vi "initializer_set_time.vi"(6 "Parameters Tree":refnum<vi>, 9 "Endtime":refnum<vi>, 10 "Starttime":refnum<vi>, 11 "Spec File Loaded?":refnum<vi>) -> ()   [LabVIEW 2019]
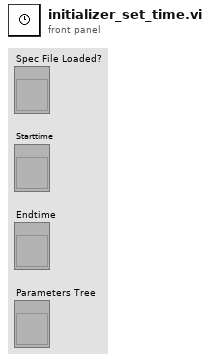
[diagram p1: front panel]
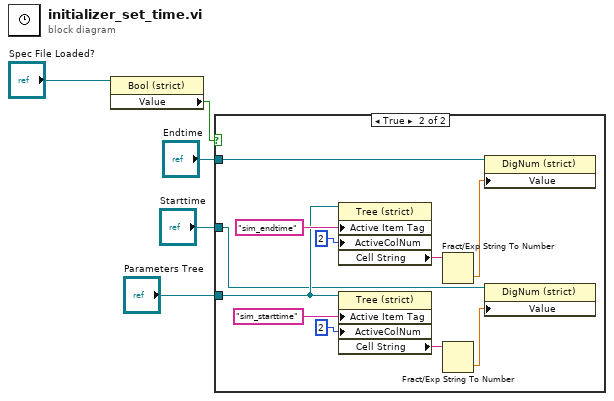
[diagram p0: block diagram]
diagram:
  n1 = property class="Bool (strict)"(reference="Spec File Loaded?") -> ("Value"=w5:bool)  [unwired: 1 in, 2 out]
  n2 = case shown="True" w5 {
    tunnel: "Parameters Tree" -> [_ w12]
    tunnel: "Starttime" -> [_ w7]
    tunnel: "Endtime" -> [_ w6]
    frame False {
    }
    frame True {
      n3 = property on="Property Node" class="Tree (strict)"(reference=w12, "Active Item Tag"="sim_endtime" ("Active Item:Tag"), "ActiveColNum"=2 ("Active Cell:Active Column Number")) -> ("Cell String"=w11:string)  [unwired: 1 in, 2 out]
      n4 = property on="Property Node" class="Tree (strict)"(reference=w12, "Active Item Tag"="sim_starttime" ("Active Item:Tag"), "ActiveColNum"=2 ("Active Cell:Active Column Number")) -> ("Cell String"=w10:string)  [unwired: 1 in, 2 out]
      n5 = Fract/Exp String To Number(string=w11) -> (number=w8:dbl)  [unwired: 3 in, 1 out]
      n6 = Fract/Exp String To Number(string=w10) -> (number=w9:dbl)  [unwired: 3 in, 1 out]
      n7 = property class="DigNum (strict)"(reference=w6, "Value"=w8) -> ()  [unwired: 1 in, 2 out]
      n8 = property class="DigNum (strict)"(reference=w7, "Value"=w9) -> ()  [unwired: 1 in, 2 out]
    }
  }
